vi "ArrayToImage.vi"(7 "image name":string="untitled", 8 "error in (no error)":errorcluster, 9 "height":i32=256, 10 "width":i32=320, 11 "image data":sgl[](array[numeric])) -> (0 "error out":errorcluster, 3 "image":T1(plugin-control))   [LabVIEW 2017]
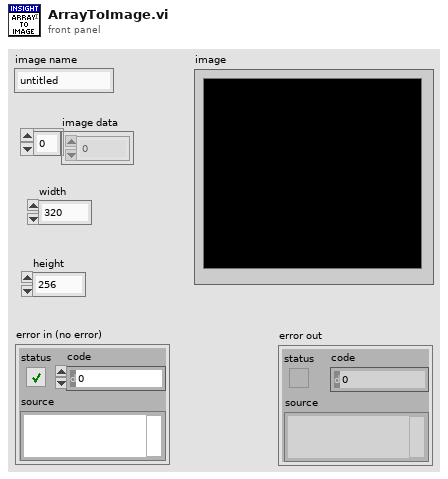
[diagram p1: front panel]
types:
  T1 = typedef "IMAQ Image.ctl" = refnum<image>
  T2 = typedef "Image Type" = u32
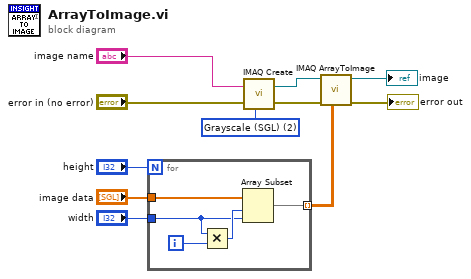
[diagram p0: block diagram]
diagram:
  w7 = T2 2 items=["Grayscale (U8)", "Grayscale (I16)", "Grayscale (SGL)", "Complex (CSG)", "RGB (U32)", "HSL (U32)", "RGB (U64)", "Grayscale (U16)"] ("Image Type")
  n1 = for {
    N: "height" -> [_]
    tunnel: "image data" -> [w16]
    tunnel: [w13] -> w10 mode=indexing
    tunnel: "width" -> [w12]
    i -> [w15]
    n2 = Multiply(x=w12, y=w15) -> (x*y=w14:i32)
    n3 = Array Subset(array=w16, index=w14, length=w12) -> (w13:sgl[])
  }
  n4 = call "IMAQ Create"("Image Name"="image name", "Image Type"=w7, "error in (no error)"="error in (no error)") -> ("New Image"=w9:T1, "error out"=w8:errorcluster)  [unwired: 2 in]
  n5 = call "IMAQ ArrayToImage"("Image Pixels (Float)"=w10, "error in (no error)"=w8, "Image"=w9) -> ("error out"=→"error out":errorcluster, "Image Out"=→"image":T1)  [unwired: 7 in]
